vi "CameraNormalizeto100.vi"(8 "error in":errorcluster, 10 "Attr String":string, 11 "IMAQdx Session in":T1) -> (0 "error out":errorcluster, 2 "Normal Value":dbl, 3 "IMAQdx Session":T1)   [LabVIEW 2025]
doc: "This VI updates an attribute where input unit is percentage and camera parameter may be in another unit.\n\nThis software is licensed. Open the labview\\readme\\WPI Robotics Library Open Source License.txt file for more information."
uses:
  <vilib>/userDefined/High Color/IMAQdx.ctl
  <resource>/objmgr/imaqdx.rc
  <vilib>/gmath/NI_Gmath.lvlib
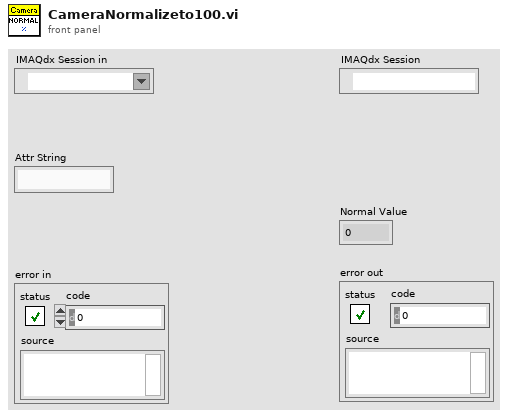
[diagram p1: front panel]
types:
  T1 = typedef "IMAQdx.ctl" = refnum<k21>
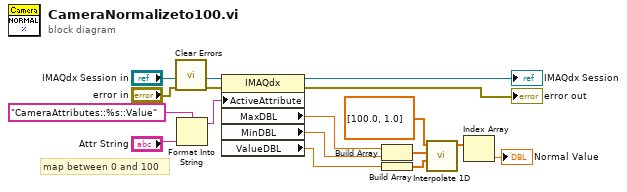
[diagram p0: block diagram]
diagram:
  # "map between 0 and 100"
  n1 = call <vilib>:"Clear Errors.vi"("error in (no error)"="error in") -> ("error out"=w6:errorcluster)  [unwired: 5 in, 1 out]
  n2 = Format Into String(format string="CameraAttributes::%s::Value" ("Attr Format"), "Attr String") -> (resulting string=w11:string)  [unwired: 2 in, 1 out]
  n3 = property class="IMAQdx"(reference="IMAQdx Session in", error in=w6, "ActiveAttribute"=w11) -> (reference out=→"IMAQdx Session":T1, error out=→"error out":errorcluster, "MaxDBL"=w2:dbl, "MinDBL"=w1:dbl, "ValueDBL"=w5:dbl)
  n4 = Build Array(w2, w1) -> (w3:dbl[])
  n5 = Build Array(w5) -> (w14:dbl[])
  n6 = call <vilib>:"Interpolate 1D.vi"("xi"=w14, "X"=w3, "Y"=dbl[] [100.0, 1.0] ("X")) -> ("yi"=w13:dbl[])  [unwired: 6 in, 2 out]
  n7 = Index Array(array=w13) -> (element=→"Normal Value":dbl)  [unwired: 1 in]
